vi "UpdateControls.vi"(8 "error in (no error)":errorcluster, 11 "Calendar in":refnum<class "Calendar.lvclass">) -> (0 "error out":errorcluster, 3 "Calendar (dup)":refnum<class "Calendar.lvclass">)   [LabVIEW 2020, in "Calendar.lvclass"]
uses:
  Calendar.lvclass
  Calendar.lvclass/Calendar.ctl
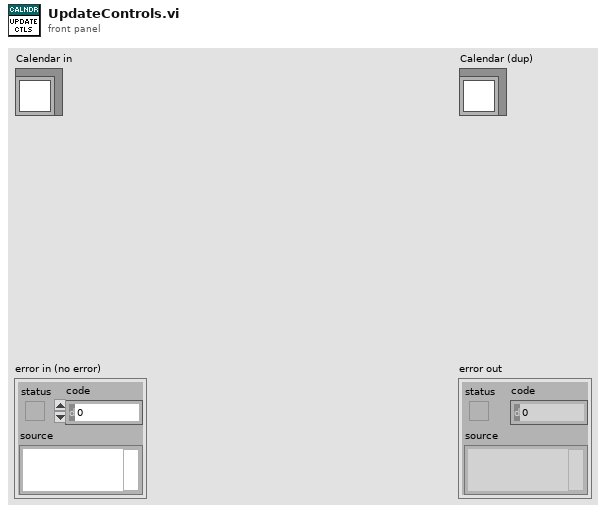
[diagram p1: front panel]
types:
  T1 = typedef "Calendar.lvclass/State Data.ctl" = cluster{"Current Date":timestamp, "First Day of Week":T2, "Color":cluster{"Selector Background":u32, "Selector Text":u32, "Days of Week Background":u32, "Days of Week Text":u32, "Calendar Background":u32, "Calendar Text":u32, "Calendar Selection Background":u32, "Calendar Selection Text":u32}, "Visible":cluster{"Today Selector Visible":bool, "Month-Year Selector Visible":bool}}
  T2 = typedef "Calendar.lvclass/DaysOfWeek.ctl" = enum16{"Sunday", "Monday", "Tuesday", "Wednesday", "Thursday", "Friday", "Saturday"}
  T3 = typedef "LVDateTimeRec.ctl" = cluster{"fractional second":dbl, "second":i32, "minute":i32, "hour":i32, "day of month":i32, "month":i32, "year":i32, "day of week":i32, "day of year":i32, "DST":i32}
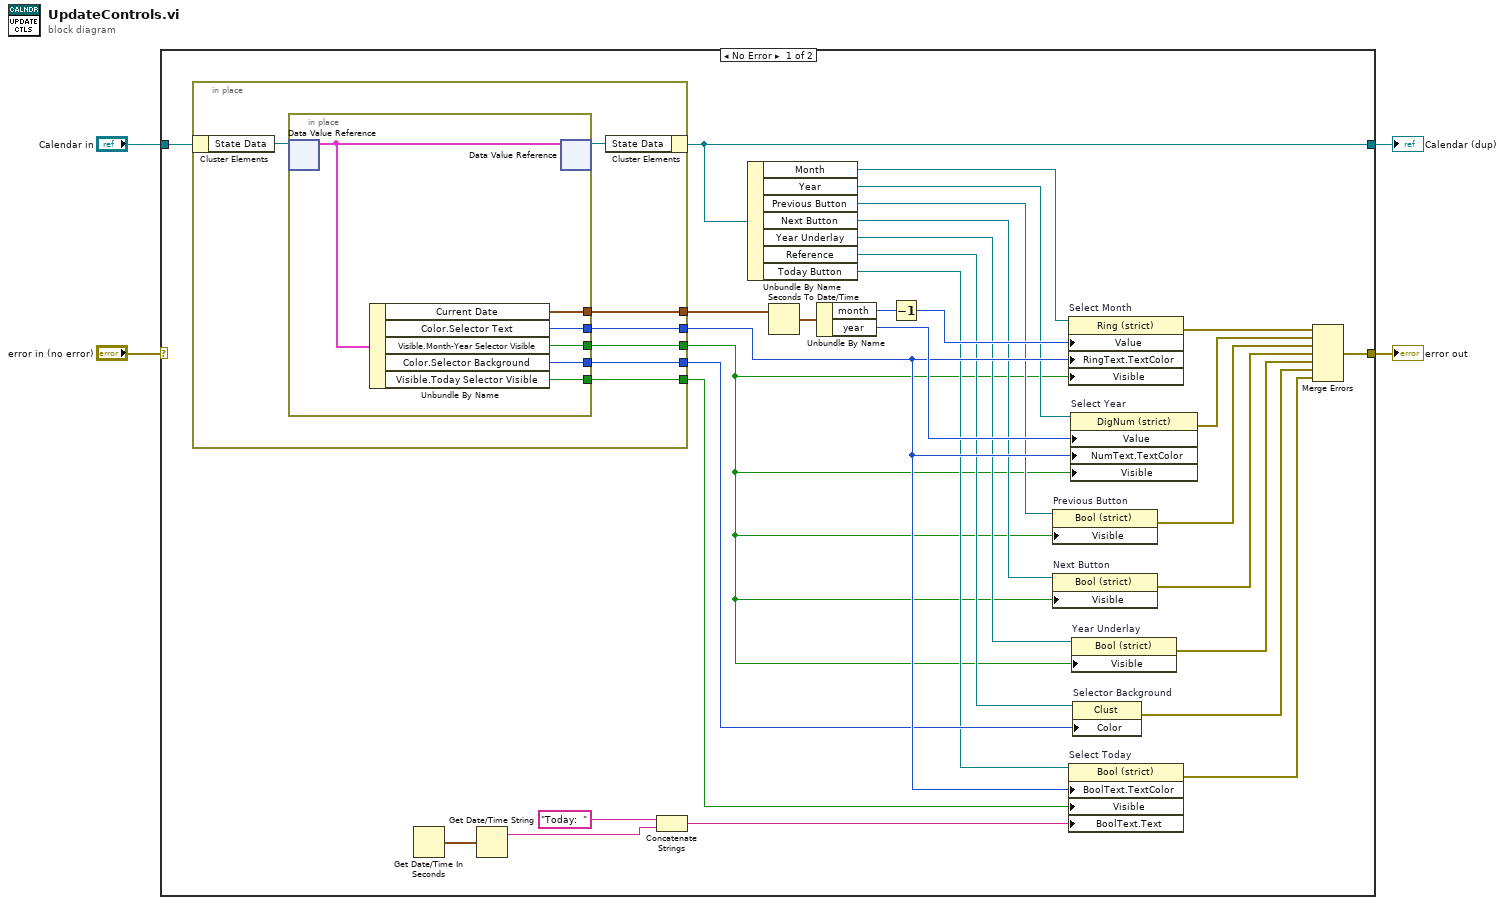
[diagram p0: block diagram]
diagram:
  n1 = case shown="No Error" "error in (no error)" {
    selector: "error in (no error)" -> [_ w49]
    tunnel: [w5 w49] -> w3
    tunnel: [w33 w48] -> w1
    tunnel: "Calendar in" -> [w34 w48]
    frame No Error {
      n2 = in-place {
        in-place-border: [w40] -> w23
        in-place-border: [w38] -> w22
        in-place-border: [w37] -> w19
        in-place-border: [w36] -> w18
        in-place-border: [w35] -> w13
        n3 = in-place-cluster #1(w34) -> ("State Data"=w41:refnum<data-value>)
        n4 = in-place {
          in-place-border: [w46] -> w40
          in-place-border: [w45] -> w38
          in-place-border: [w44] -> w37
          in-place-border: [w43] -> w36
          in-place-border: [w42] -> w35
          n5 = in-place-dvr #2(w41) -> (w47:T1)  [unwired: 1 out]
          n6 = Unbundle By Name(w47) -> ("Current Date"=w46:timestamp, "Color.Selector Text"=w45:u32, "Visible.Month-Year Selector Visible"=w42:bool, "Color.Selector Background"=w44:u32, "Visible.Today Selector Visible"=w43:bool)
          n7 = in-place-dvr #2(w47) -> (w39:refnum<data-value>)  [unwired: 1 out]
        }
        n8 = in-place-cluster #1("State Data"=w39) -> (w33:refnum<class "Calendar.lvclass">)
      }
      n9 = Get Date/Time In Seconds() -> (seconds since 1Jan1904=w28:timestamp)
      n10 = Get Date/Time String(seconds (now)=w28) -> (date string=w27:string)  [unwired: 2 in, 1 out]
      n11 = Concatenate Strings("Today:  " ("Boolean Text.Text"), w27) -> (w26:string)
      n12 = Unbundle By Name(w33) -> ("Month"=w24:refnum<vi>, "Year"=w21:refnum<vi>, "Previous Button"=w16:refnum<vi>, "Next Button"=w15:refnum<vi>, "Year Underlay"=w14:refnum<vi>, "Reference"=w20:refnum<vi>, "Today Button"=w17:refnum<vi>)
      n13 = Seconds To Date/Time(time stamp (now)=w23) -> (date time rec=w29:T3)  [unwired: 1 out]
      n14 = Unbundle By Name(w29) -> ("month"=w30:i32, "year"=w32:i32)
      n15 = Decrement(x=w30) -> (x-1=w31:i32)
      n16 = property on="Previous Button" class="Bool (strict)"(reference=w16, "Visible"=w13) -> (error out=w10:errorcluster)  [unwired: 1 in, 1 out]
      n17 = property on="Next Button" class="Bool (strict)"(reference=w15, "Visible"=w13) -> (error out=w9:errorcluster)  [unwired: 1 in, 1 out]
      n18 = property on="Select Month" class="Ring (strict)"(reference=w24, "Value"=w31, "RingText.TextColor"=w22, "Visible"=w13) -> (error out=w12:errorcluster)  [unwired: 1 in, 1 out]
      n19 = property on="Select Today" class="Bool (strict)"(reference=w17, "BoolText.TextColor"=w22, "Visible"=w18, "BoolText.Text"=w26) -> (error out=w6:errorcluster)  [unwired: 1 in, 1 out]
      n20 = property on="Select Year" class="DigNum (strict)"(reference=w21, "Value"=w32, "NumText.TextColor"=w22, "Visible"=w13) -> (error out=w11:errorcluster)  [unwired: 1 in, 1 out]
      n21 = property on="Year Underlay" class="Bool (strict)"(reference=w14, "Visible"=w13) -> (error out=w8:errorcluster)  [unwired: 1 in, 1 out]
      n22 = property on="Selector Background" class="Clust"(reference=w20, "Color"=w19) -> (error out=w7:errorcluster)  [unwired: 1 in, 1 out]
      n23 = Merge Errors(w12, w11, w10, w9, w8, w7, w6) -> (w5:errorcluster)
    }
    frame Error {
    }
  }
  "error out" <- w3
  "Calendar (dup)" <- w1
